vi "UI.vi"() -> ()   [LabVIEW 2020]
uses:
  <vilib>/LabVIEW Interface for Arduino/Type Defs/Pin Mode.ctl
  <vilib>/LabVIEW Interface for Arduino/Type Defs/Board Type.ctl
  <vilib>/LabVIEW Interface for Arduino/Type Defs/Connection Type.ctl
  9cd75f8d-94f0-4fab-b97a-d62b9cef563f.vi
  <vilib>/LabVIEW Interface for Arduino/LabVIEW Interface for Arduino.lvlib
panel:
  out "Waveform Chart":i16(graph)
  out "RPM":i16
  in  "stop":bool
  in  "Duty Cycle (0 - 255)":u8(knob) scale=0.0..254.0
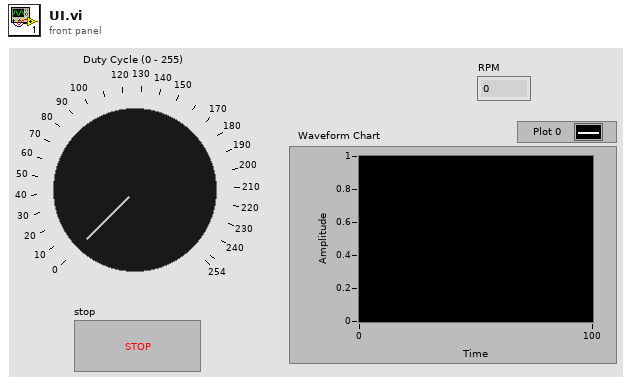
[diagram p1: front panel]
types:
  T1 = typedef "LabVIEW Interface for Arduino.lvlib/Connection Type.ctl" = enum8{"USB / Serial", "XBEE", "BlueSmirf (Bluetooth)"}
  T2 = typedef "LabVIEW Interface for Arduino.lvlib/Board Type.ctl" = enum16{"Uno", "Dimuelanove w/Atmega 328", "Mega 2560"}
  T3 = typedef "LabVIEW Interface for Arduino.lvlib/Pin Mode.ctl" = enum8{"Input", "Output"}
  T4 = typedef "LabVIEW Interface for Arduino.lvlib/Arduino Resource.ctl" = cluster{"VISA resource":refnum<visa-resource-name>, "Board Type":T2, "Connection Type":enum8{"USB / Serial"}, "Bytes Per Packet (15)":u8}
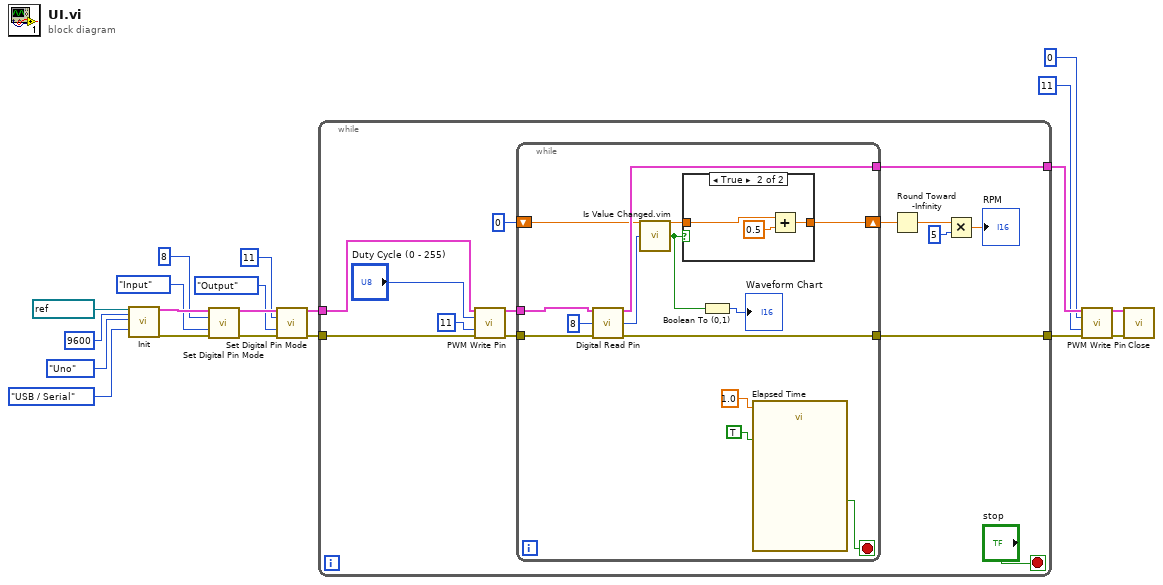
[diagram p0: block diagram]
diagram:
  n1 = call <vilib>:"Init.vi"("VISA resource"=refnum<visa-resource-name> "COM6", "Baud Rate (115200)"=u32 9600, "Board Type (Uno)"=Board_Type."Uno", "Connection Type (USB/Serial)"=Connection_Type."USB / Serial") -> ("Arduino Resource"=w20:T4, "error out"=w19:errorcluster)  [unwired: 14 in]
  n2 = call <vilib>:"Set Digital Pin Mode.vi"("Arduino Resource"=w20, "Digital I/O Pin"=u8 8, "Pin Mode (Input)"=Pin_Mode."Input", "error in"=w19) -> ("Arduino Resource"=w16:T4, "error out"=w15:errorcluster)  [unwired: 10 in]
  n3 = call <vilib>:"Set Digital Pin Mode.vi"("Arduino Resource"=w16, "Digital I/O Pin"=u8 11, "Pin Mode (Input)"=Pin_Mode."Output", "error in"=w15) -> ("Arduino Resource"=w12:T4, "error out"=w11:errorcluster)  [unwired: 10 in]
  n4 = while {
    tunnel: w12 -> [w34]
    tunnel: w11 -> [w33]
    tunnel: [w25] -> w6
    tunnel: [w24] -> w5
    stop <- "stop" stop-if-true
    n5 = call <vilib>:"PWM Write Pin.vi"("Arduino Resource"=w34, "Duty Cycle (0 - 255)"="Duty Cycle (0 - 255)", "PWM Pin (3)"=u8 11, "error in"=w33) -> ("Arduino Resource"=w27:T4, "error out"=w26:errorcluster)  [unwired: 10 in]
    n6 = while {
      tunnel: w27 -> [w47]
      tunnel: w26 -> [w46]
      tunnel: [w44] -> w25
      tunnel: [w43] -> w24
      shift-right: [w41] -> w22
      shift-left: u8 0 -> [w42]
      stop <- w39 stop-if-true
      n7 = call <vilib>:"Digital Read Pin.vi"("Arduino Resource"=w47, "Digital I/O Pin (0)"=u8 8, "error in"=w46) -> ("Arduino Resource"=w44:T4, "Value"=w37:u8, "error out"=w43:errorcluster)  [unwired: 10 in]
      n8 = call "Is Value Changed.vim"("value"=w37) -> ("changed or first call?"=w36:bool)
      n9 = case shown="True" w36 {
        tunnel: w42 -> [w48 w51]
        tunnel: [w48 w50] -> w41
        frame False {
        }
        frame True {
          n10 = Add(x=w51, y=0.5) -> (x+y=w50:dbl)
        }
      }
      n11 = Boolean To (0,1)(Boolean=w36) -> (0, 1=→"Waveform Chart":i16)
      n12 = call "Elapsed Time"("Time Target (s)"=1.0, "Auto Reset"=TRUE) -> ("Time has Elapsed"=w39:bool)  [unwired: 10 in, 7 out]
    }
    n13 = Round Toward -Infinity(1:w22) -> (0:w21:dbl)
    n14 = Multiply(x=w21, y=u8 5) -> (x*y=→"RPM":dbl)
  }
  n15 = call <vilib>:"PWM Write Pin.vi"("Arduino Resource"=w6, "Duty Cycle (0 - 255)"=u8 0, "PWM Pin (3)"=u8 11, "error in"=w5) -> ("Arduino Resource"=w3:T4, "error out"=w4:errorcluster)  [unwired: 10 in]
  n16 = call <vilib>:"Close.vi"("Arduino Resource"=w3, "error in"=w4) -> ()  [unwired: 13 in, 1 out]
